vi "PH_SHS_Analysis.Zernike Coefficient Names.vi"() -> (0 "Zernickes":string[](array[string]))   [LabVIEW 2014, in "PH_SHS_Analysis.lvlib"]
doc: "This VI gets the names of the Zernicke coefficients."
uses:
  PH_SHS_Analysis.lvlib
  PH_SHS_Analysis.Zernike Coefficients.ctl
panel:
  in  "Zernike Coefficients":T1 {"2nd Spherical" scale=-2.0..2.0 scale format="%.2f"; "2nd Coma y" scale=-2.0..2.0 scale format="%.2f"; "2nd Coma x" scale=-2.0..2.0 scale format="%.2f"; "2nd Astig 45°" scale=-2.0..2.0 scale format="%.2f"; "2nd Astig 0°" scale=-2.0..2.0 scale format="%.2f"; "Trefoil 30°" scale=-2.0..2.0 scale format="%.2f"; "Trefoil 0°" scale=-2.0..2.0 scale format="%.2f"; "Spherical" scale=-2.0..2.0 scale format="%.2f"; "Coma y" scale=-2.0..2.0 scale format="%.2f"; "Coma x" scale=-2.0..2.0 scale format="%.2f"; "Astig 45°" scale=-2.0..2.0 scale format="%.2f"; "Astig 0°" scale=-2.0..2.0 scale format="%.2f"; "Defocus" scale=-2.0..2.0 scale format="%.2f"; "Tilt y" scale=-2.0..2.0 scale format="%.2f"; "Tilt x" scale=-2.0..2.0 scale format="%.2f"}
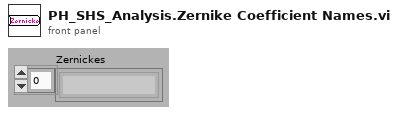
[diagram p1: front panel]
types:
  T1 = typedef "PH_SHS_Analysis.lvlib/PH_SHS_Analysis.Zernike Coefficients.ctl" = cluster{"Tilt x":dbl, "Tilt y":dbl, "Defocus":dbl, "Astig 0°":dbl, "Astig 45°":dbl, "Coma x":dbl, "Coma y":dbl, "Spherical":dbl, "Trefoil 0°":dbl, "Trefoil 30°":dbl, "2nd Astig 0°":dbl, "2nd Astig 45°":dbl, "2nd Coma x":dbl, "2nd Coma y":dbl, "2nd Spherical":dbl}
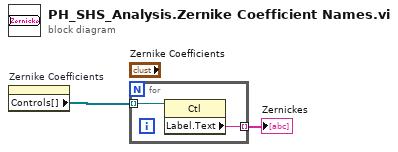
[diagram p0: block diagram]
diagram:
  n1 = property on="Zernike Coefficients" class="Clust (strict)"() -> ("Controls[]"=w1:refnum<vi>[])  [unwired: 2 in, 2 out]
  n2 = for {
    tunnel: [w4] -> w2 mode=indexing
    tunnel: w1 -> [w3] mode=indexing
    n3 = property class="Ctl"(reference=w3) -> ("Label.Text"=w4:string)  [unwired: 1 in, 2 out]
  }
  "Zernickes" <- w2
